vi "While Loop SCTL Benchmarking.vi"() -> ()   [LabVIEW 2012]
panel:
  out "Avg Ticks (SCTL)":u32
  out "Ticks (SCTL)":u32
  out "Avg Ticks (While Loop)":u32
  out "Ticks (While Loop)":u32
  in  "Value A":i16
  in  "Value B":i16
  in  "Value C":i16
  in  "Value D":i16
  out "Average Value (ABCD)":i16
  in  "Value 1":i16
  in  "Value 2":i16
  in  "Value 3":i16
  in  "Value 4":i16
  out "Average Value (1234)":i16
  # "While Loop Benchmark"
  # "SCTL Benchmark"
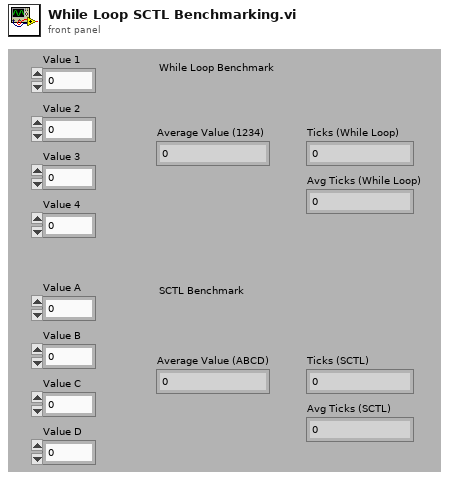
[diagram p1: front panel]
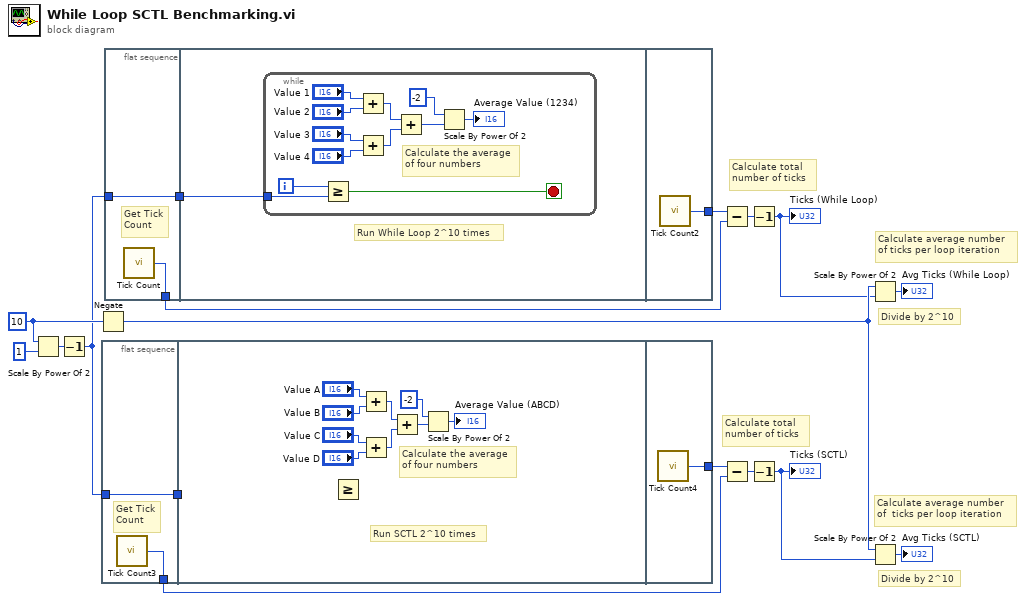
[diagram p0: block diagram]
diagram:
  w13 = 10 ("n")
  # "Calculate total\nnumber of ticks"
  # "Calculate total\nnumber of ticks"
  # "Calculate average number\nof  ticks per loop iteration"
  # "Divide by 2^10"
  # "Divide by 2^10"
  # "Calculate average number\nof ticks per loop iteration"
  n1 = Scale By Power Of 2(n=w13, x=1) -> (x*2^n=w14:i32)
  n2 = Decrement(x=w14) -> (x-1=w12:i32)
  n3 = Negate(x=w13) -> (-x=w7:i32)
  n4 = flat-sequence {
    tunnel: [w19] -> w16
    tunnel: w12 -> [w19]
    tunnel: [w18] -> w5
    tunnel: w16 -> [_]
    tunnel: [w29] -> w6
    frame #0 {
      # "Get Tick\nCount"
      n5 = call "Tick Count3"() -> ("Tick Count(Ticks)"=w18:u32)
    }
    frame #1 {
      # "Calculate the average\nof four numbers"
      # "Run SCTL 2^10 times"
      n6 = Greater Or Equal?() -> ()  [unwired: 2 in, 1 out]
      n7 = Add(x="Value A", y="Value B") -> (x+y=w24:i16)
      n8 = Add(x="Value C", y="Value D") -> (x+y=w23:i16)
      n9 = Add(x=w24, y=w23) -> (x+y=w21:i16)
      n10 = Scale By Power Of 2(n=-2, x=w21) -> (x*2^n=→"Average Value (ABCD)":i16)
    }
    frame #2 {
      n11 = call "Tick Count4"() -> ("Tick Count(Ticks)"=w29:u32)
    }
  }
  n12 = flat-sequence {
    tunnel: w12 -> [w31]
    tunnel: [w31] -> w17
    tunnel: [w30] -> w10
    tunnel: w17 -> [w32]
    tunnel: [w45] -> w9
    frame #0 {
      # "Get Tick\nCount"
      n13 = call "Tick Count"() -> ("Tick Count(Ticks)"=w30:u32)
    }
    frame #1 {
      # "Run While Loop 2^10 times"
      n14 = while {
        tunnel: w32 -> [w33]
        i -> [w44]
        stop <- w43 stop-if-true
        # "Calculate the average\nof four numbers"
        n15 = Greater Or Equal?(x=w44, y=w33) -> (x >= y?=w43:bool)
        n16 = Add(x="Value 1", y="Value 2") -> (x+y=w38:i16)
        n17 = Add(x="Value 3", y="Value 4") -> (x+y=w37:i16)
        n18 = Add(x=w38, y=w37) -> (x+y=w35:i16)
        n19 = Scale By Power Of 2(n=-2, x=w35) -> (x*2^n=→"Average Value (1234)":i16)
      }
    }
    frame #2 {
      n20 = call "Tick Count2"() -> ("Tick Count(Ticks)"=w45:u32)
    }
  }
  n21 = Subtract(x=w9, y=w10) -> (x-y=w4:u32)
  n22 = Subtract(x=w6, y=w5) -> (x-y=w2:u32)
  n23 = Decrement(x=w4) -> (x-1=w3:u32)
  "Ticks (While Loop)" <- w3
  n24 = Decrement(x=w2) -> (x-1=w1:u32)
  "Ticks (SCTL)" <- w1
  n25 = Scale By Power Of 2(n=w7, x=w3) -> (x*2^n=→"Avg Ticks (While Loop)":u32)
  n26 = Scale By Power Of 2(n=w7, x=w1) -> (x*2^n=→"Avg Ticks (SCTL)":u32)
